vi "Q8381 Check Wavelength Prm.vi"(1 "Unit":u16(ring) items=["um ", "nm"], 2 "Wavelength":dbl=1.55 format="%.6f") -> (0 "GPIB Status":bool)   [LabVIEW 2017]
doc: "Wavelength\n um : 0.35 - 1.75\n nm : 350 - 1750"
panel:
  # "Check Wavelength Parameter"
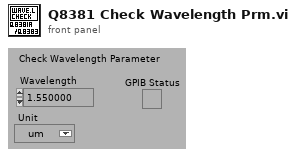
[diagram p1: front panel]
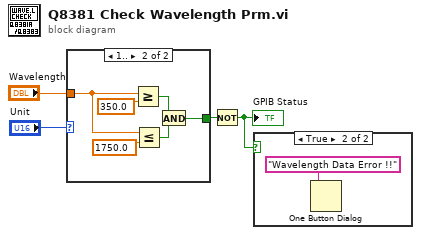
[diagram p0: block diagram]
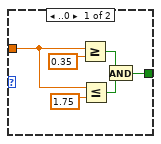
[diagram p3: hidden frame]
diagram:
  n1 = case shown="1.." "Unit" {
    tunnel: "Wavelength" -> [w10 w12]
    tunnel: [w5 w11] -> w2
    frame ..0 {
      n2 = Greater Or Equal?(x=w10, y=0.35) -> (x >= y?=w7:bool)
      n3 = Less Or Equal?(x=w10, y=1.75) -> (x <= y?=w6:bool)
      n4 = And(x=w7, y=w6) -> (x .and. y?=w5:bool)
    }
    frame 1.. {
      n5 = Greater Or Equal?(x=w12, y=350.0) -> (x >= y?=w14:bool)
      n6 = Less Or Equal?(x=w12, y=1750.0) -> (x <= y?=w13:bool)
      n7 = And(x=w14, y=w13) -> (x .and. y?=w11:bool)
    }
  }
  n8 = Not(x=w2) -> (.not. x?=w1:bool)
  "GPIB Status" <- w1
  n9 = case shown="True" w1 {
    frame False {
    }
    frame True {
      n10 = One Button Dialog(message="Wavelength Data Error !!") -> ()  [unwired: 1 in, 1 out]
    }
  }
